vi "Parse To Type.vi"(7 "Type and Defaults":variant, 8 "error in (no error)":errorcluster, 10 "Variant in":variant, 11 "Deserializer in":refnum<class "JSON Deserializer.lvclass">) -> (0 "error out":errorcluster, 2 "Variant out":variant, 3 "Deserializer out":refnum<class "JSON Deserializer.lvclass">)   [LabVIEW 2013, in "JKI JSON Serialization.lvlib" / "JSON Deserializer.lvclass"]
doc: "JKI Serialization 1.0.0.4\nTomi Maila - JKI\nCopyright (c) 2016, JKI"
uses:
  JSON Deserializer.lvclass
  <vilib>/Utility/VariantDataType/VariantType.lvlib
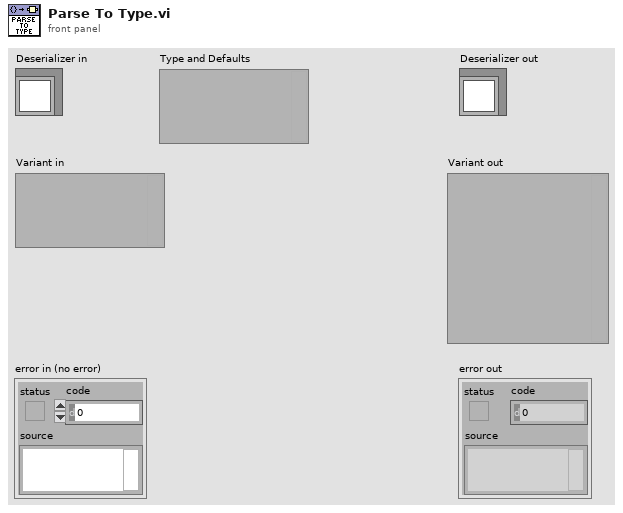
[diagram p1: front panel]
types:
  T1 = typedef "VariantType.lvlib/Type.ctl" = enum8{"Invalid Type", "Void", "I8", "I16", "I32", "I64", "U8", "U16", "U32", "U64", "Single Float", "Double Float", "Extended Float", "Single Complex", "Double Complex", "Extended Complex", "Enum U8", "Enum U16", "Enum U32", "Enum U64", "Single Float With Unit", "Double Float With Unit", "Extended Float With Unit", "Single Complex with Unit", "Double Complex with Unit", "Extended Complex with Unit", "Boolean", "String", "Path", "Picture", "Tag", "Array", "Cluster", "Variant", "LV Variant", "Waveform", "Timestamp", "Digital Waveform", "Digital Data", "ExpressData", "Refnum", "External Data", "VI", "Poly VI", "LabVIEW Class Instance", "Fixed Point"}
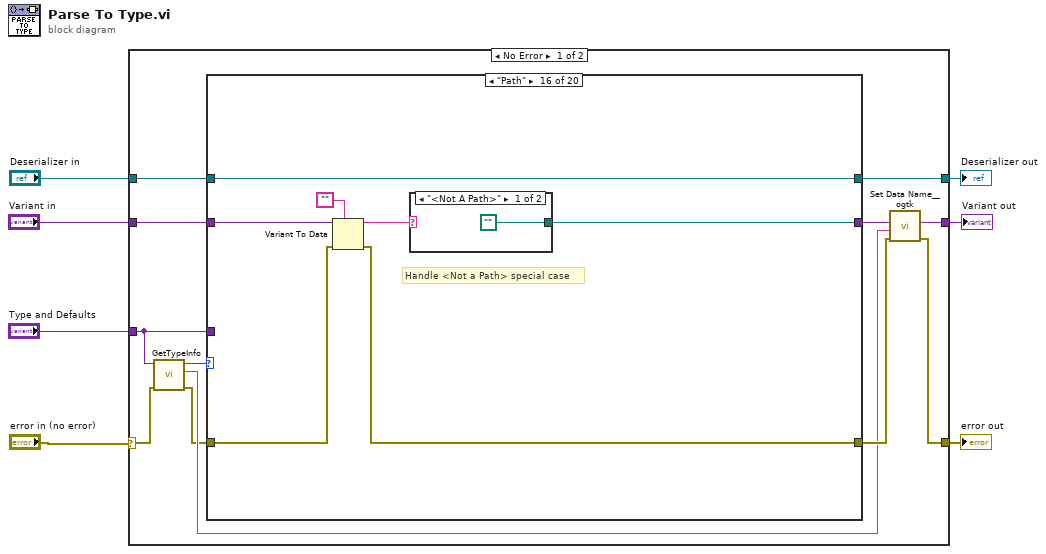
[diagram p0: block diagram]
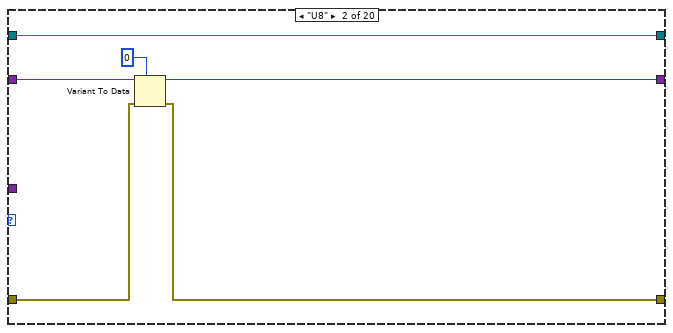
[diagram p3: hidden frame]
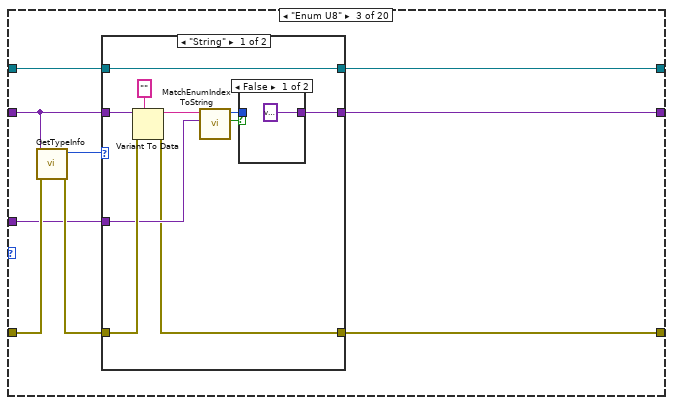
[diagram p4: hidden frame]
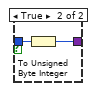
[diagram p5: hidden frame]
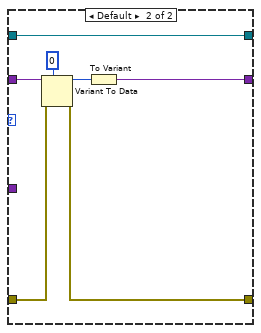
[diagram p6: hidden frame]
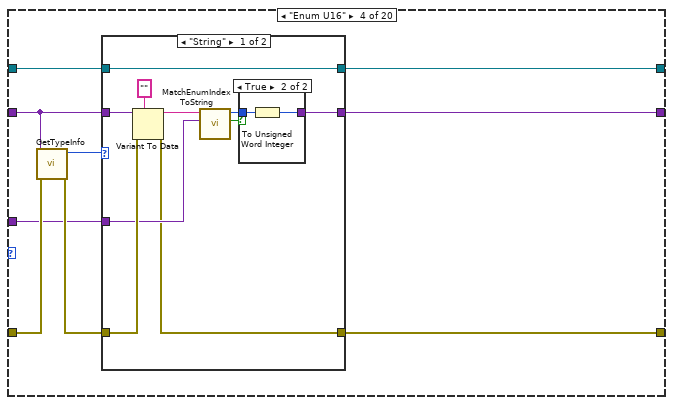
[diagram p7: hidden frame]
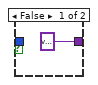
[diagram p8: hidden frame]
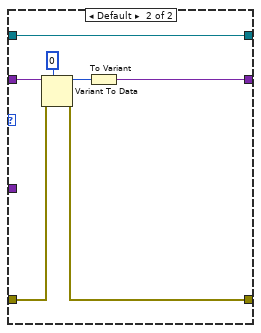
[diagram p9: hidden frame]
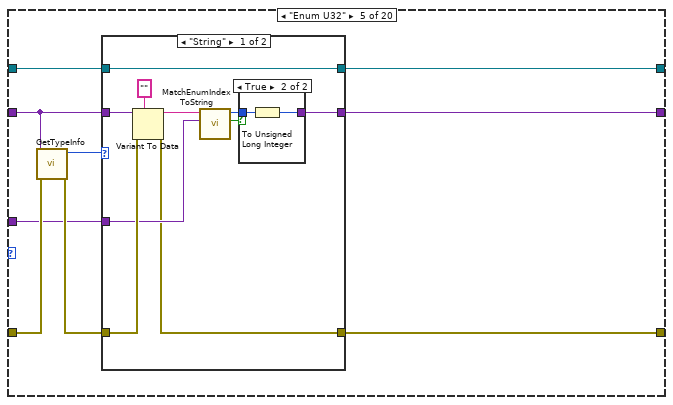
[diagram p10: hidden frame]
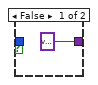
[diagram p11: hidden frame]
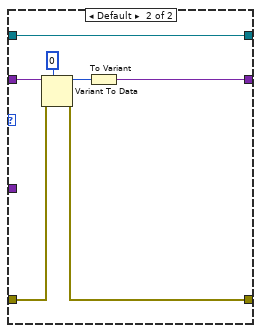
[diagram p12: hidden frame]
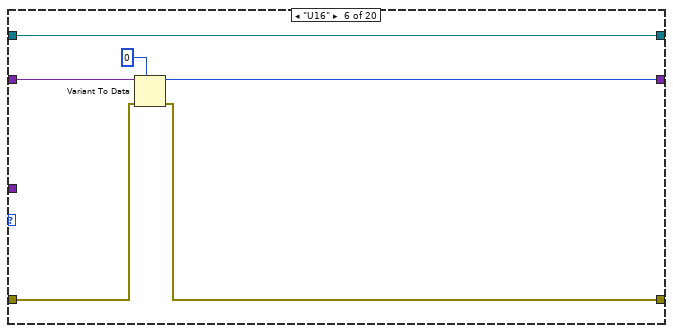
[diagram p13: hidden frame]
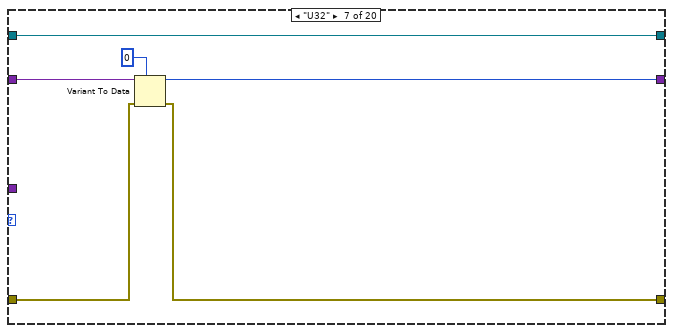
[diagram p14: hidden frame]
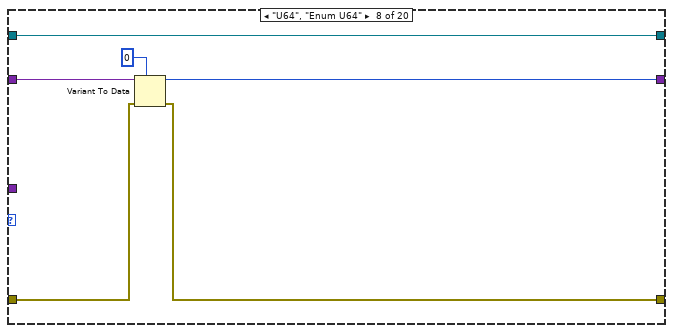
[diagram p15: hidden frame]
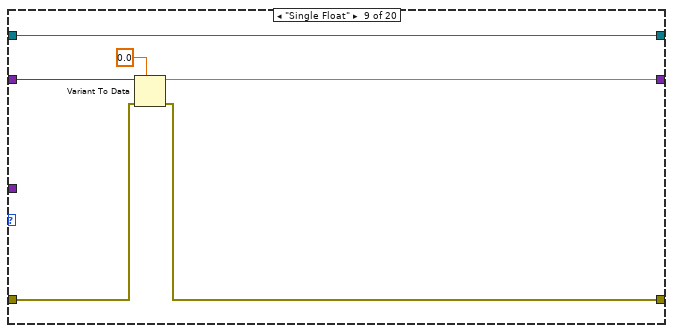
[diagram p16: hidden frame]
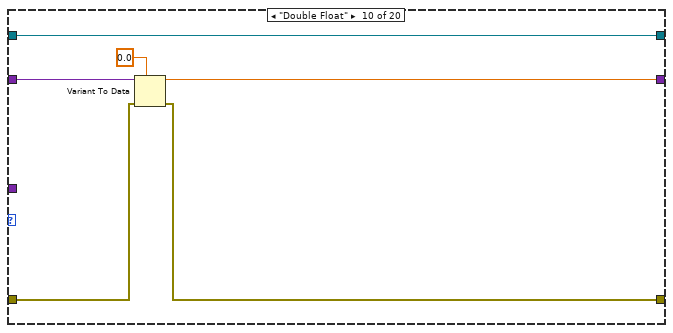
[diagram p17: hidden frame]
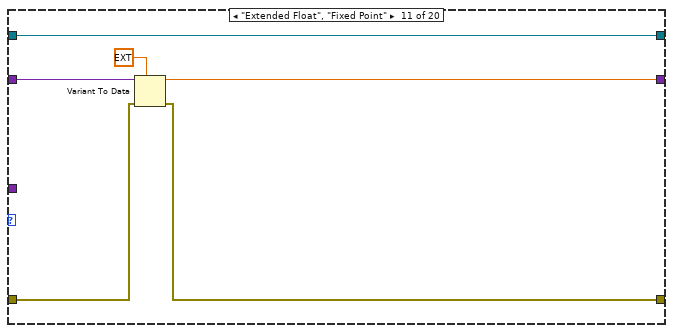
[diagram p18: hidden frame]
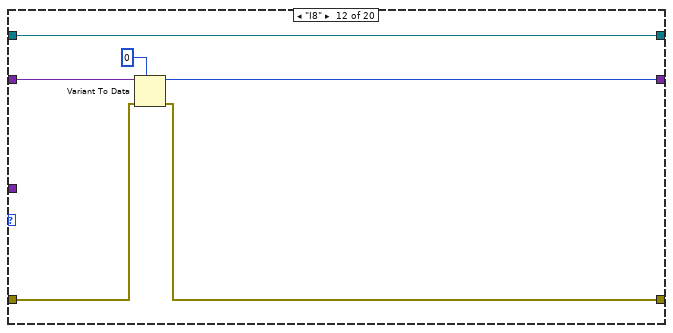
[diagram p19: hidden frame]
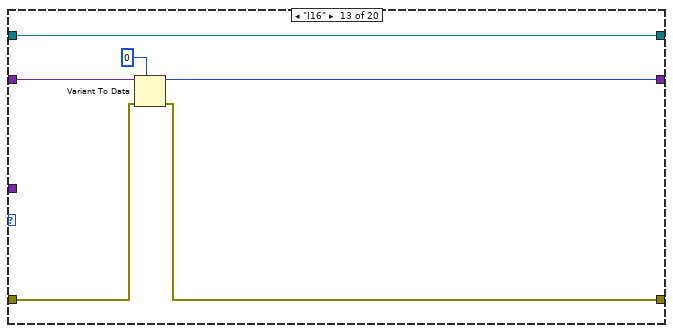
[diagram p20: hidden frame]
diagram:
  n1 = case shown="No Error" "error in (no error)" {
    selector: "error in (no error)" -> [w16 w343]
    tunnel: "Deserializer in" -> [w18 w344]
    tunnel: "Variant in" -> [w14 _]
    tunnel: [w11 w343] -> w4
    tunnel: "Type and Defaults" -> [w15 w342]
    tunnel: [w17 w344] -> w2
    tunnel: [w12 w342] -> w1
    frame No Error {
      n2 = call <vilib>:"GetTypeInfo.vi"("error in (no error)"=w16, "Variant"=w15) -> ("error out"=w8:errorcluster, "Name"=w9:string, "Type Enum"=w19:T1)  [unwired: 5 in, 2 out]
      n3 = case shown="\"Path\"" w19 {
        tunnel: [w21 w25 w35 w64 w93 w118 w124 w130 w136 w142 w148 w154 w160 w166 w172 w179 w187 w200 w259 w339] -> w10
        tunnel: w8 -> [w21 w26 w33 w62 w91 w119 w125 w131 w137 w143 w149 w155 w161 w167 w173 w180 w191 w202 w258 w340]
        tunnel: w18 -> [w22 w28 w31 w60 w89 w121 w127 w133 w139 w145 w151 w157 w163 w169 w175 w182 w193 w199 w263 w341]
        tunnel: [w22 w28 w30 w59 w88 w121 w127 w133 w139 w145 w151 w157 w163 w169 w175 w182 w193 w197 w262 w341] -> w17
        tunnel: w15 -> [_ _ w29 w58 w87 _ _ _ _ _ _ _ _ _ _ _ _ w203 w261 _]
        tunnel: w14 -> [w20 w27 w36 w65 w94 w120 w126 w132 w138 w144 w150 w156 w162 w168 w174 w181 w192 w194 w256 w338]
        tunnel: [w20 w23 w37 w66 w95 w116 w122 w128 w134 w140 w146 w152 w158 w164 w170 w177 w186 w196 w260 w338] -> w13
        frame "Void", Default {
        }
        frame "U8" {
          n4 = Variant To Data(error in=w26, type=u8 0, Variant=w27) -> (data=w23:u8, error out=w25:errorcluster)
        }
        frame "Enum U8" {
          n5 = call <vilib>:"GetTypeInfo.vi"("error in (no error)"=w33, "Variant"=w36) -> ("error out"=w32:errorcluster, "Type Enum"=w34:T1)  [unwired: 5 in, 3 out]
          n6 = case shown="\"String\"" w34 {
            tunnel: [w41 w51] -> w37
            tunnel: w36 -> [w47 w55]
            tunnel: w32 -> [w45 w54]
            tunnel: [w38 w53] -> w35
            tunnel: w31 -> [w39 w52]
            tunnel: [w39 w52] -> w30
            tunnel: w29 -> [w43 _]
            frame "String" {
              n7 = Variant To Data(error in=w45, type="", Variant=w47) -> (data=w44:string, error out=w38:errorcluster)
              n8 = call "MatchEnumIndexToString.vi"("Enum Variant"=w43, "String"=w44) -> ("found"=w40:bool, "index"=w42:i32)  [unwired: 8 in]
              n9 = case shown="False" w40 {
                tunnel: w42 -> [_ w50]
                tunnel: [variant ("Type and Defaults") w49] -> w41
                frame False {
                }
                frame True {
                  n10 = To Unsigned Byte Integer(number=w50) -> (unsigned 8bit integer=w49:u8)
                }
              }
            }
            frame Default {
              n11 = Variant To Data(error in=w54, type=u8 0, Variant=w55) -> (data=w56:u8, error out=w53:errorcluster)
              n12 = To Variant(anything=w56) -> (Variant=w51:variant)
            }
          }
        }
        frame "Enum U16" {
          n13 = call <vilib>:"GetTypeInfo.vi"("error in (no error)"=w62, "Variant"=w65) -> ("error out"=w61:errorcluster, "Type Enum"=w63:T1)  [unwired: 5 in, 3 out]
          n14 = case shown="\"String\"" w63 {
            tunnel: [w70 w80] -> w66
            tunnel: w65 -> [w76 w84]
            tunnel: w61 -> [w74 w83]
            tunnel: [w67 w82] -> w64
            tunnel: w60 -> [w68 w81]
            tunnel: [w68 w81] -> w59
            tunnel: w58 -> [w72 _]
            frame "String" {
              n15 = Variant To Data(error in=w74, type="", Variant=w76) -> (data=w73:string, error out=w67:errorcluster)
              n16 = call "MatchEnumIndexToString.vi"("Enum Variant"=w72, "String"=w73) -> ("found"=w69:bool, "index"=w71:i32)  [unwired: 8 in]
              n17 = case shown="True" w69 {
                tunnel: w71 -> [_ w79]
                tunnel: [variant ("Type and Defaults") w78] -> w70
                frame False {
                }
                frame True {
                  n18 = To Unsigned Word Integer(number=w79) -> (unsigned 16bit integer=w78:u16)
                }
              }
            }
            frame Default {
              n19 = Variant To Data(error in=w83, type=u16 0, Variant=w84) -> (data=w85:u16, error out=w82:errorcluster)
              n20 = To Variant(anything=w85) -> (Variant=w80:variant)
            }
          }
        }
        frame "Enum U32" {
          n21 = call <vilib>:"GetTypeInfo.vi"("error in (no error)"=w91, "Variant"=w94) -> ("error out"=w90:errorcluster, "Type Enum"=w92:T1)  [unwired: 5 in, 3 out]
          n22 = case shown="\"String\"" w92 {
            tunnel: [w99 w109] -> w95
            tunnel: w94 -> [w105 w113]
            tunnel: w90 -> [w103 w112]
            tunnel: [w96 w111] -> w93
            tunnel: w89 -> [w97 w110]
            tunnel: [w97 w110] -> w88
            tunnel: w87 -> [w101 _]
            frame "String" {
              n23 = Variant To Data(error in=w103, type="", Variant=w105) -> (data=w102:string, error out=w96:errorcluster)
              n24 = call "MatchEnumIndexToString.vi"("Enum Variant"=w101, "String"=w102) -> ("found"=w98:bool, "index"=w100:i32)  [unwired: 8 in]
              n25 = case shown="True" w98 {
                tunnel: w100 -> [_ w108]
                tunnel: [variant ("Type and Defaults") w107] -> w99
                frame False {
                }
                frame True {
                  n26 = To Unsigned Long Integer(number=w108) -> (unsigned 32bit integer=w107:u32)
                }
              }
            }
            frame Default {
              n27 = Variant To Data(error in=w112, type=u32 0, Variant=w113) -> (data=w114:u32, error out=w111:errorcluster)
              n28 = To Variant(anything=w114) -> (Variant=w109:variant)
            }
          }
        }
        frame "U16" {
          n29 = Variant To Data(error in=w119, type=u16 0, Variant=w120) -> (data=w116:u16, error out=w118:errorcluster)
        }
        frame "U32" {
          n30 = Variant To Data(error in=w125, type=u32 0, Variant=w126) -> (data=w122:u32, error out=w124:errorcluster)
        }
        frame "U64", "Enum U64" {
          n31 = Variant To Data(error in=w131, type=u64 0, Variant=w132) -> (data=w128:u64, error out=w130:errorcluster)
        }
        frame "Single Float" {
          n32 = Variant To Data(error in=w137, type=sgl 0.0, Variant=w138) -> (data=w134:sgl, error out=w136:errorcluster)
        }
        frame "Double Float" {
          n33 = Variant To Data(error in=w143, type=0.0, Variant=w144) -> (data=w140:dbl, error out=w142:errorcluster)
        }
        frame "Extended Float", "Fixed Point" {
          n34 = Variant To Data(error in=w149, type=ext 0.0, Variant=w150) -> (data=w146:ext, error out=w148:errorcluster)
        }
        frame "I8" {
          n35 = Variant To Data(error in=w155, type=i8 0, Variant=w156) -> (data=w152:i8, error out=w154:errorcluster)
        }
        frame "I16" {
          n36 = Variant To Data(error in=w161, type=i16 0, Variant=w162) -> (data=w158:i16, error out=w160:errorcluster)
        }
        frame "I32" {
          n37 = Variant To Data(error in=w167, type=0, Variant=w168) -> (data=w164:i32, error out=w166:errorcluster)
        }
        frame "I64" {
          n38 = Variant To Data(error in=w173, type=i64 0, Variant=w174) -> (data=w170:i64, error out=w172:errorcluster)
        }
        frame "Path" {
          # "Handle <Not a Path> special case"
          n39 = Variant To Data(error in=w180, type="", Variant=w181) -> (data=w176:string, error out=w179:errorcluster)
          n40 = case shown="\"<Not A Path>\"" w176 {
            selector: w176 -> [_ w184]
            tunnel: [path "" w185] -> w177
            frame "<Not A Path>" {
            }
            frame Default {
              n41 = String To Path(string=w184) -> (path=w185:path)
            }
          }
        }
        frame "Timestamp" {
          n42 = Variant To Data(error in=w191, type="", Variant=w192) -> (data=w189:string, error out=w188:errorcluster)
          n43 = call "ISO String To Timestamp.vi"("error in (no error)"=w188, "ISO Timestamp String"=w189) -> ("error out"=w187:errorcluster, "Time Stamp"=w186:timestamp)  [unwired: 8 in]
        }
        frame "Array" {
          n44 = call <vilib>:"GetArrayInfo.vi"("error in (no error)"=w202, "Variant"=w203) -> ("error out"=w201:errorcluster, "ArrayElement"=w198:variant, "NDims"=w195:i32)  [unwired: 6 in, 1 out]
          n45 = case shown="1" w195 {
            tunnel: w201 -> [w206 w213]
            tunnel: w194 -> [w208 w211]
            tunnel: [w207 w218] -> w200
            tunnel: w199 -> [w209 w217]
            tunnel: w198 -> [_ w216]
            tunnel: [w209 w215] -> w197
            tunnel: [w208 w214] -> w196
            frame 2, Default {
              n46 = call <vilib>:"Error Cluster From Error Code.vi"("error in (no error)"=w206, "error message (\"\")"="Unflattening failed. Multidimensional arrays not supported." ("error message (\"\")"), "error code (0)"=1) -> ("error out"=w207:errorcluster)  [unwired: 6 in]
            }
            frame 1 {
              n47 = call <vilib>:"GetTypeInfo.vi"("error in (no error)"=w213, "Variant"=w211) -> ("error out"=w212:errorcluster, "Type Enum"=w210:T1)  [unwired: 5 in, 3 out]
              n48 = case shown="\"Cluster\"" w210 {
                tunnel: [w219 w229 w247] -> w218
                tunnel: w217 -> [w221 w227 w246]
                tunnel: w216 -> [w220 w226 w245]
                tunnel: [w221 w225 w244] -> w215
                tunnel: [w220 w224 w243] -> w214
                tunnel: w212 -> [w219 w223 w240]
                tunnel: w211 -> [_ w222 w242]
                frame Default {
                }
                frame "Array" {
                  n49 = Variant To Data(error in=w223, type=variant[] [], Variant=w222) -> (data=w230:variant[], error out=w228:errorcluster)
                  n50 = for {
                    tunnel: w230 -> [w237] mode=indexing
                    shift-right: [w235] -> w229
                    shift-left: w228 -> [w236]
                    shift-right: [w233] -> w225
                    shift-left: w227 -> [w238]
                    tunnel: w226 -> [w234]
                    tunnel: [w232] -> w224 mode=indexing
                    n51 = call "Parse To Type.vi"("Type and Defaults"=w234, "error in (no error)"=w236, "Variant in"=w237, "Deserializer in"=w238) -> ("error out"=w235:errorcluster, "Variant out"=w232:variant, "Deserializer out"=w233:refnum<class "JSON Deserializer.lvclass">)  [unwired: 5 in]
                  }
                }
                frame "Cluster" {
                  n52 = call <userlib>:"Cluster to Array of VData__ogtk.vi"("error in (no error)"=w240, "Cluster"=w242) -> ("error out"=w241:errorcluster, "Array of VData"=w239:variant[])  [unwired: 8 in]
                  n53 = for {
                    tunnel: w239 -> [w253] mode=indexing
                    shift-right: [w251] -> w247
                    shift-left: w241 -> [w252]
                    shift-right: [w249] -> w244
                    shift-left: w246 -> [w254]
                    tunnel: w245 -> [w250]
                    tunnel: [w248] -> w243 mode=indexing
                    n54 = call "Parse To Type.vi"("Type and Defaults"=w250, "error in (no error)"=w252, "Variant in"=w253, "Deserializer in"=w254) -> ("error out"=w251:errorcluster, "Variant out"=w248:variant, "Deserializer out"=w249:refnum<class "JSON Deserializer.lvclass">)  [unwired: 5 in]
                  }
                }
              }
            }
          }
        }
        frame "Cluster" {
          n55 = call <vilib>:"GetTypeInfo.vi"("error in (no error)"=w258, "Variant"=w256) -> ("error out"=w257:errorcluster, "Type Enum"=w255:T1)  [unwired: 5 in, 3 out]
          n56 = case shown="\"Void\"" w255 {
            tunnel: w263 -> [w269 w272 w278 w310]
            tunnel: [w269 w272 w277 w309] -> w262
            tunnel: w261 -> [w268 w271 w284 w308]
            tunnel: [w268 w271 w275 w300] -> w260
            tunnel: [w267 w270 w273 w297] -> w259
            tunnel: w257 -> [w266 w270 w283 w296]
            tunnel: w256 -> [_ _ w285 w295]
            frame "Invalid Type", Default {
              n57 = call <vilib>:"Error Cluster From Error Code.vi"("error in (no error)"=w266, "error message (\"\")"="Cannot deserialize the input type into a cluster." ("error message (\"\")"), "error code (0)"=1) -> ("error out"=w267:errorcluster)  [unwired: 6 in]
            }
            frame "Void" {
              # "Empty input object, use default values"
            }
            frame "Array" {
              n58 = call <userlib>:"Cluster to Array of VData__ogtk.vi"("error in (no error)"=w283, "Cluster"=w284) -> ("error out"=w282:errorcluster, "Array of VData"=w281:variant[])  [unwired: 8 in]
              n59 = call <userlib>:"Array to Array of VData__ogtk.vi"("error in (no error)"=w282, "MultiD Array"=w285) -> ("error out"=w279:errorcluster, "1D Array of Variants"=w280:variant[])  [unwired: 8 in]
              n60 = for {
                tunnel: w281 -> [w290] mode=indexing
                tunnel: w280 -> [w293]
                shift-right: [w288] -> w274
                shift-left: w279 -> [w289]
                shift-right: [w287] -> w277
                shift-left: w278 -> [w294]
                tunnel: [w286] -> w276 mode=indexing
                i -> [w292]
                n61 = Index Array(array=w293, index=w292) -> (element=w291:variant)
                n62 = call "Parse To Type.vi"("Type and Defaults"=w290, "error in (no error)"=w289, "Variant in"=w291, "Deserializer in"=w294) -> ("error out"=w288:errorcluster, "Variant out"=w286:variant, "Deserializer out"=w287:refnum<class "JSON Deserializer.lvclass">)  [unwired: 5 in]
              }
              n63 = call <userlib>:"Array of VData to VCluster__ogtk.vi"("error in (no error)"=w274, "Array"=w276) -> ("error out"=w273:errorcluster, "VCluster"=w275:variant)  [unwired: 8 in]
            }
            frame "Cluster" {
              n64 = call <userlib>:"Cluster to Array of VData__ogtk.vi"("error in (no error)"=w296, "Cluster"=w308) -> ("error out"=w306:errorcluster, "Array of VData"=w307:variant[])  [unwired: 8 in]
              n65 = call <userlib>:"Cluster to Array of VData__ogtk.vi"("error in (no error)"=w306, "Cluster"=w295) -> ("error out"=w302:errorcluster, "Array of VData"=w305:variant[])  [unwired: 8 in]
              n66 = for {
                tunnel: w305 -> [w312] mode=indexing
                shift-right: [w313] -> w301
                shift-left: w302 -> [w314]
                tunnel: [w312] -> w304 mode=indexing
                tunnel: [w311] -> w303 mode=indexing
                n67 = call <vilib>:"GetTypeInfo.vi"("error in (no error)"=w314, "Variant"=w312) -> ("error out"=w313:errorcluster, "Name"=w311:string)  [unwired: 5 in, 3 out]
              }
              n68 = for {
                shift-right: [w324] -> w298
                shift-left: w301 -> [w319]
                shift-right: [w323] -> w309
                shift-left: w310 -> [w325]
                tunnel: w307 -> [w316] mode=indexing
                tunnel: [w322] -> w299 mode=indexing
                tunnel: w304 -> [w317]
                tunnel: w303 -> [w321]
                n69 = call <vilib>:"GetTypeInfo.vi"("error in (no error)"=w319, "Variant"=w316) -> ("error out"=w318:errorcluster, "Name"=w320:string)  [unwired: 5 in, 3 out]
                n70 = Search 1D Array(1D array=w321, element=w320) -> (index of element=w315:i32)  [unwired: 1 in]
                n71 = case shown="0.." w315 {
                  selector: w315 -> [_ w329]
                  tunnel: w325 -> [w328 w337]
                  tunnel: [w326 w336] -> w324
                  tunnel: [w328 w335] -> w323
                  tunnel: [w327 w334] -> w322
                  tunnel: w318 -> [w326 w333]
                  tunnel: w317 -> [_ w332]
                  tunnel: w316 -> [w327 w330]
                  frame ..-1 {
                    # "Element not found"
                  }
                  frame 0.. {
                    # "Element found"
                    n72 = Index Array(array=w332, index=w329) -> (element=w331:variant)
                    n73 = call "Parse To Type.vi"("Type and Defaults"=w330, "error in (no error)"=w333, "Variant in"=w331, "Deserializer in"=w337) -> ("error out"=w336:errorcluster, "Variant out"=w334:variant, "Deserializer out"=w335:refnum<class "JSON Deserializer.lvclass">)  [unwired: 5 in]
                  }
                }
              }
              n74 = call <userlib>:"Array of VData to VCluster__ogtk.vi"("error in (no error)"=w298, "Array"=w299) -> ("error out"=w297:errorcluster, "VCluster"=w300:variant)  [unwired: 8 in]
            }
          }
        }
        frame "LV Variant" {
          # "Empty input object, use default values"
          n75 = call <vilib>:"GetTypeInfo.vi"("error in (no error)"=w340, "Variant"=w338) -> ("error out"=w339:errorcluster)  [unwired: 5 in, 4 out]
        }
      }
      n76 = call <userlib>:"Set Data Name__ogtk.vi"("error in (no error)"=w10, "Data Name"=w9, "Data"=w13) -> ("error out"=w11:errorcluster, "Renamed Data"=w12:variant)  [unwired: 7 in]
    }
    frame Error {
    }
  }
  "error out" <- w4
  "Deserializer out" <- w2
  "Variant out" <- w1
